vi "OPC UA Client.vi"() -> ()   [LabVIEW 2018]
uses:
  <vilib>/OPCUA/controls/NodeIds.ctl
  <vilib>/OPCUA/controls/NodeId.ctl
  <vilib>/OPCUA/client/Multiple Read UInt64.vi
  <vilib>/OPCUA/NI OPC UA Client.lvlib
panel:
  out "Frequency":u64
  in  "stop":bool
  out "error out":errorcluster
  in  "Server endpoint URL":string
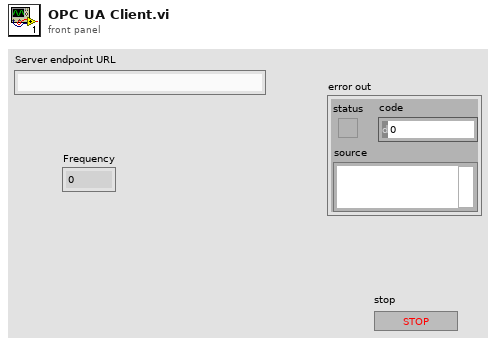
[diagram p1: front panel]
types:
  T1 = typedef "OPC UA Client Refnum.ctl" = refnum<k21>
  T2 = typedef "NodeIds.ctl" = T3[]
  T3 = typedef "NodeId.ctl" = string
  T4 = typedef "OPC UA StatusCode.ctl" = u32
  T5 = cluster{"node ID":T3, "value ":u64, "timestamp":timestamp, "status":T4}[]
  T6 = cluster{"node ID":T3, "value ":u64, "timestamp":timestamp, "status":T4}
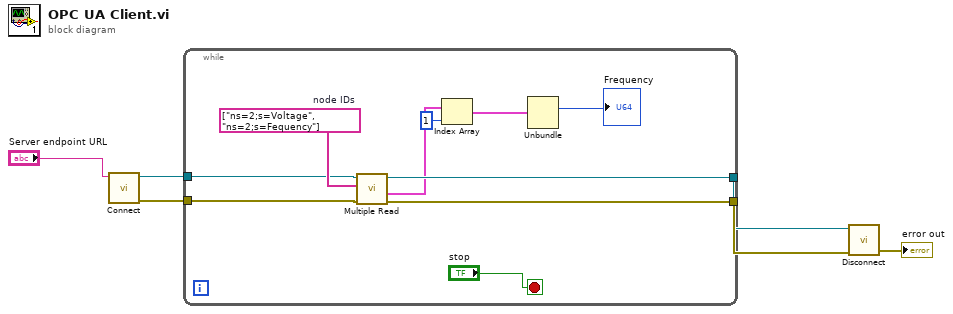
[diagram p0: block diagram]
diagram:
  n1 = call <vilib>:"Connect.vi"("server endpoint URL"="Server endpoint URL") -> ("error out"=w3:errorcluster, "OPC UA client refnum out"=w4:T1)  [unwired: 8 in, 1 out]
  n2 = while {
    tunnel: w4 -> [w14]
    tunnel: w3 -> [w13]
    tunnel: [w12] -> w2
    tunnel: [w11] -> w1
    stop <- "stop" stop-if-true
    w15 = T2 ["ns=2;s=Voltage", "ns=2;s=Fequency"]  # node IDs
    n3 = call-poly <vilib>:"Multiple Read.vi"("error in (no error)"=w13, "node IDs"=w15, "OPC UA client refnum in"=w14) -> ("error out"=w12:errorcluster, "results"=w10:T5, "OPC UA client refnum out"=w11:T1)  [unwired: 5 in, 1 out]
    n4 = Index Array(array=w10, index=1) -> (element=w9:T6)
    n5 = Unbundle(w9) -> ("value"=→"Frequency":u64)  [unwired: 3 out]
  }
  n6 = call <vilib>:"Disconnect.vi"("error in (no error)"=w2, "OPC UA client refnum in"=w1) -> ("error out"=→"error out":errorcluster)  [unwired: 9 in]
